vi "Agilent 34420 Read Triggered Multiple.vi"() -> ()   [LabVIEW 2021]
doc: "This example shows how to configure a measurement, set up triggering, trigger a measurement, and retrieve a measurement. It shows how to use the low-level Data VIs to retrieve data from the 34420."
uses:
  <instrlib>/Agilent 34420/Agilent 34420.lvlib
panel:
  in  "Sample Count (1)":i32=1 format="%#.6g"
  in  "Trigger Count (1)":i32=1 format="%#.6g"
  in  "Function (0: DC Volts)":u16(ring) items=["DC Volts", "DC Voltage Ratio", "DC Voltage Difference", "2 Wire Resistance", "4 Wire Resistance", "Temperature"]
  in  "Serial Configuration":T1={"Baud Rate"=9600, "Parity"=0, "Data Bits"=8} {"Data Bits" items=["7"=7, "8"=8]; "Parity" items=["None", "Odd", "Even", "Mark", "Space"]; "Baud Rate" items=["300"=300, "600"=600, "1200"=1200, "2400"=2400, "4800"=4800, "9600"=9600]}
  in  "Timeout (20000 ms)":u32=20000
  out "Waveform Chart":dbl[](graph)
  in  "VISA resource name":refnum<visa-resource-name>
  # "(c) 2008-2015 National Instruments Corp.  ALL RIGHTS RESERVED."
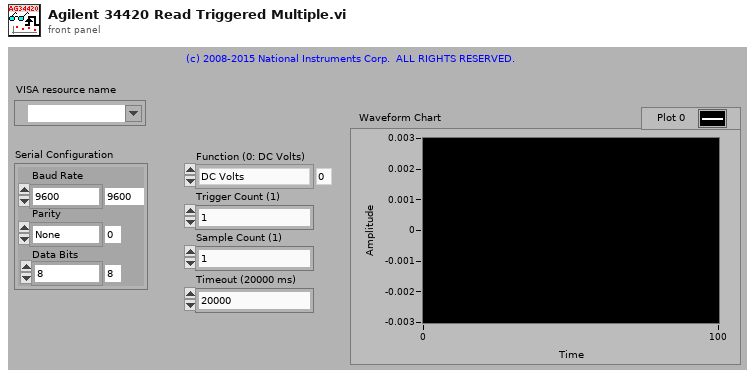
[diagram p1: front panel]
types:
  T1 = cluster{"Baud Rate":u32, "Parity":u16, "Data Bits":u16}
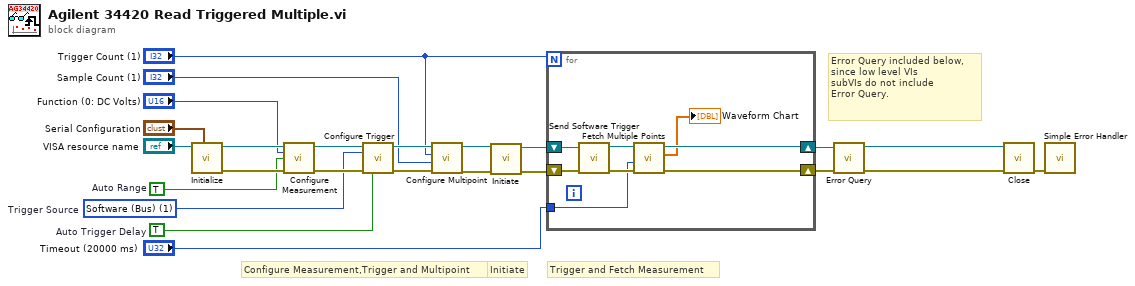
[diagram p0: block diagram]
diagram:
  w13 = u16 1 items=["Immediate", "Software (Bus)", "External"]  # Trigger Source
  w14 = TRUE  # Auto Range
  w15 = TRUE  # Auto Trigger Delay
  # "Error Query included below, \nsince low level VIs \nsubVIs do not include \nError Query."
  # "Trigger and Fetch Measurement"
  # "Initiate"
  # "Configure Measurement,Trigger and Multipoint"
  n1 = call <instrlib>:"Initialize.vi"("Serial Configuration"="Serial Configuration", "VISA resource name"="VISA resource name") -> ("error out"=w22:errorcluster, "VISA resource name out"=w23:refnum<visa-resource-name>)  [unwired: 8 in]
  n2 = call <instrlib>:"Configure Measurement.vi"("VISA resource name"=w23, "Function (0: DC Volts)"="Function (0: DC Volts)", "Auto Range (T:Enable)"=w14, "error in (no error)"=w22) -> ("VISA resource name out"=w21:refnum<visa-resource-name>, "error out"=w20:errorcluster)  [unwired: 10 in]
  n3 = call <instrlib>:"Configure Trigger.vi"("VISA resource name"=w21, "Trigger Source (0: Immediate)"=w13, "error in (no error)"=w20, "Auto Trigger Delay (T:Enable)"=w15) -> ("VISA resource name out"=w19:refnum<visa-resource-name>, "error out"=w18:errorcluster)  [unwired: 10 in]
  n4 = call <instrlib>:"Configure Multipoint.vi"("error in (no error)"=w18, "Sample Count (1)"="Sample Count (1)", "Trigger Count (1)"="Trigger Count (1)", "VISA resource name"=w19) -> ("error out"=w11:errorcluster, "VISA resource name out"=w12:refnum<visa-resource-name>)  [unwired: 6 in]
  n5 = call <instrlib>:"Initiate.vi"("error in (no error)"=w11, "VISA resource name"=w12) -> ("error out"=w10:errorcluster, "VISA resource name out"=w9:refnum<visa-resource-name>)  [unwired: 8 in]
  n6 = for {
    N: "Trigger Count (1)" -> [_]
    shift-right: [w31] -> w6
    shift-left: w10 -> [w26]
    tunnel: "Timeout (20000 ms)" -> [w25]
    shift-right: [w32] -> w8
    shift-left: w9 -> [w27]
    n7 = call <instrlib>:"Send Software Trigger.vi"("error in (no error)"=w26, "VISA resource name"=w27) -> ("error out"=w28:errorcluster, "VISA resource name out"=w29:refnum<visa-resource-name>)  [unwired: 8 in]
    n8 = call <instrlib>:"Fetch Multiple Points.vi"("error in (no error)"=w28, "Timeout (20000 ms)"=w25, "VISA resource name"=w29) -> ("error out"=w31:errorcluster, "Measurements"=→"Waveform Chart":dbl[], "VISA resource name out"=w32:refnum<visa-resource-name>)  [unwired: 6 in]
  }
  n9 = call <instrlib>:"Error Query.vi"("error in (no error)"=w6, "VISA resource name"=w8) -> ("error out"=w5:errorcluster, "VISA resource name out"=w7:refnum<visa-resource-name>)  [unwired: 6 in, 2 out]
  n10 = call <instrlib>:"Close.vi"("error in (no error)"=w5, "VISA resource name"=w7) -> ("error out"=w17:errorcluster)  [unwired: 9 in]
  n11 = call <vilib>:"Simple Error Handler.vi"("error in (no error)"=w17) -> ()  [unwired: 4 in, 5 out]
